vi "FGGA Serial Data Server & Recordingv4.3_10Hz.vi"(0 "VISA resource name out":refnum<visa-resource-name>, 11 "error IO":errorcluster) -> ()   [LabVIEW 2014]
uses:
  <vilib>/Instr/_visa.llb/VISA Configure Serial Port (Instr).vi
  <vilib>/Platform/TimedLoop/XDataNode/wakeup.ctl
  <vilib>/Platform/TimedLoop/XDataNode/XDNodeRunTimeDep.lvlib
  <vilib>/Platform/TimedLoop/XDataNode/nitl_modes.ctl
  <vilib>/Platform/TimedLoop/XDataNode/timing_clust.ctl
  <vilib>/platform/TimedLoop/XDataNode/XDataNode.xnode
  <vilib>/Utility/tcp.llb/UDP Multicast Write-Only Open.vi
  <vilib>/Utility/error.llb/whitespace.ctl
  C:/Program Files (x86)/National Instruments/LabVIEW 2014/examples/Data Communication/Network Streams/Simple Network Streams/support/Network Stream Command.ctl
panel:
  out "FGGA Pump":bool
  out "Flight Number":string
  out "Stop File Write":bool
  out "Default file name":string
  out "MFC":dbl[](array[numeric])
  out "FGGA restart":bool
  out "V4":bool
  out "V3":bool
  out "V2":bool
  out "V1":bool
  out "error out 2":errorcluster
  out "error out":errorcluster
  in  "MFC_1 SLPM set value":dbl
  out "Value Read":string
  out "status":bool
  in  "VISA resource name":refnum<visa-resource-name>="ASRL3::INSTR"
  in  "timeout (10sec) 2":u32=3000
  out "Labview_Viewer_UDP_Error_Out":errorcluster
  in  "Clear Display\nErrors":bool
  out "Data Processing":bool
  out "TCP Binary Packet":string
  out "UDP Time Stamp Offset":i32=1
  out "Data String":string
  out "UDP_ACSII_Out":string
  out "Serial error out":errorcluster
  out "SEPTIC TCP Error Out":errorcluster
  out "TCP packet\nSend To SEPTIC":bool
  out "FISH TCP Error Out":errorcluster
  out "TCP packet\nSend To FISH":bool
  out "UDP_Pack_num":u32
  out "UDP_Out Status":bool
  out "UDP_Out_Error Out":errorcluster
  out "Data Array":string[](array[string])
  out "RAW DATA":string
  in  "stop":bool
  out "Number of times \nRead time out":u32
  out "Loop count":i32
  # "Date"
  # "Time"
  # "CH4"
  # "CO2"
  # "H2O"
  # "Cell Pressure"
  # "Cell Temperature"
  # "Spectral Flag"
  # "Ring Down Time (Laser A)"
  # "Ring Down Time (Laser B)"
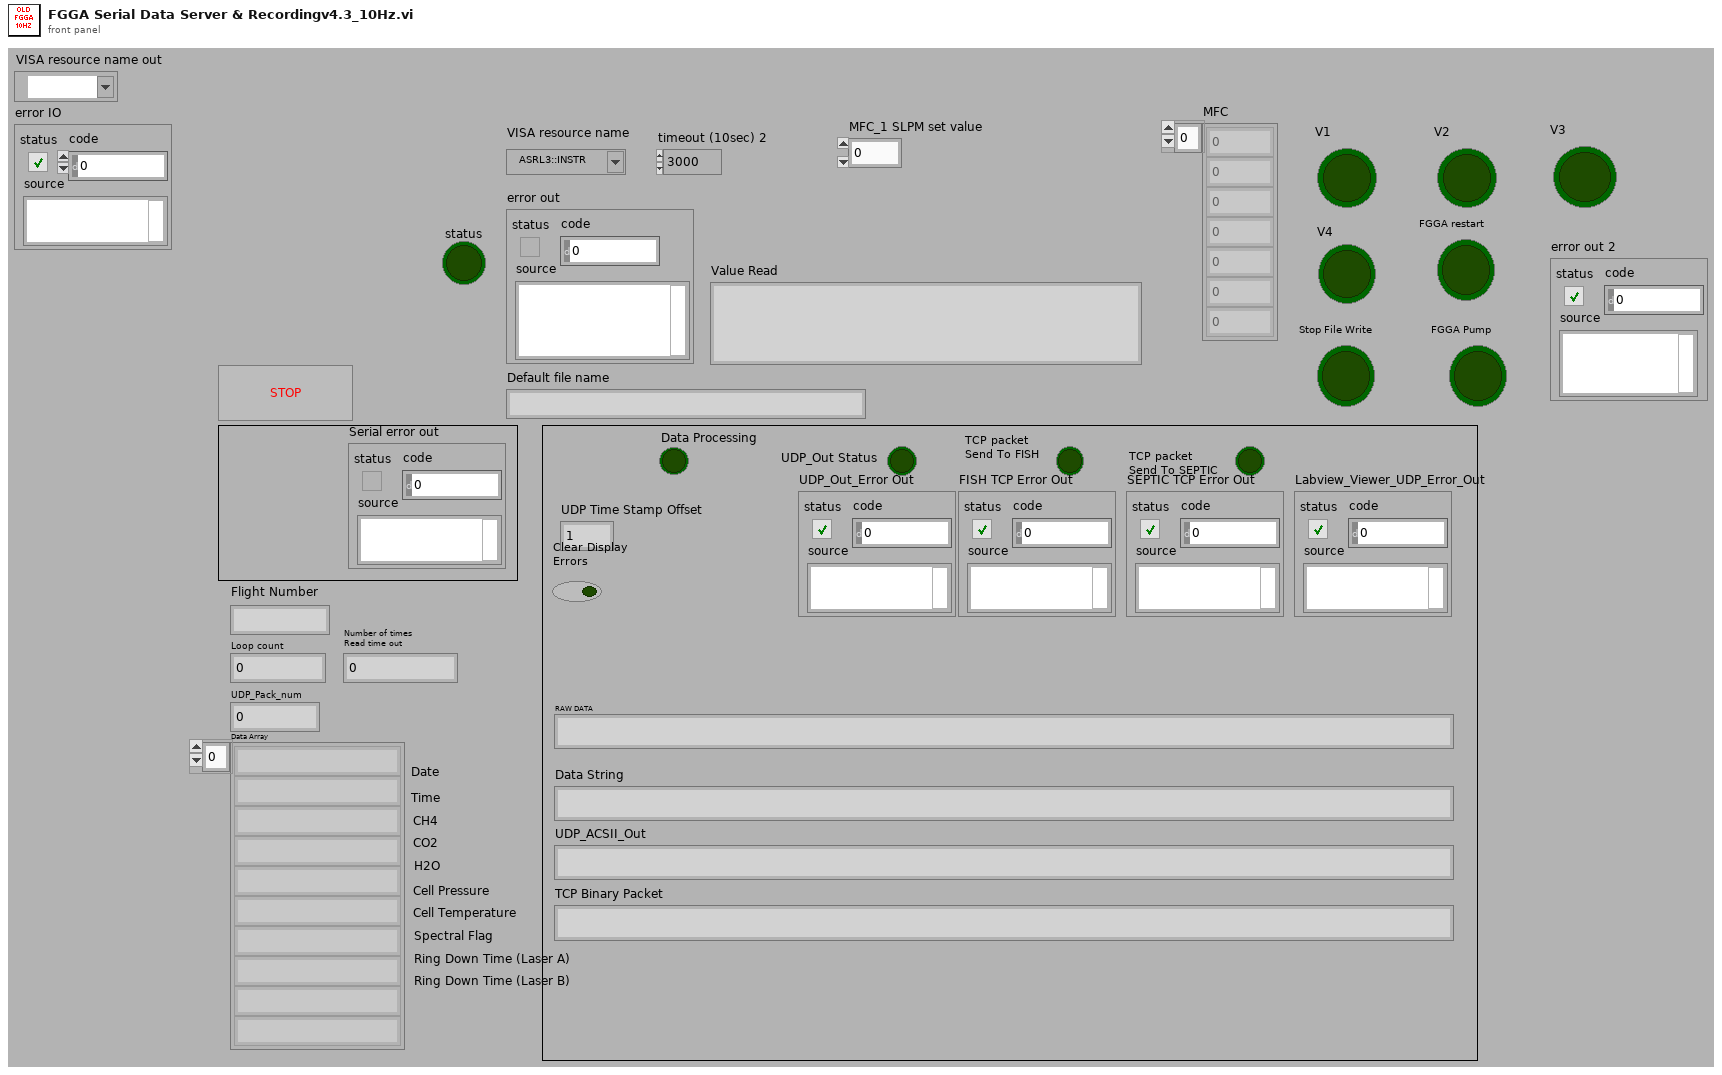
[diagram p1: front panel]
types:
  T1 = typedef "XDNodeRunTimeDep.lvlib/timing_clust.ctl" = cluster{"Expected End [f-1]":u64, "Actual End [f-1]":u64, "Finished Late? [f-1]":bool, "Expected End [i-1]":u64, "Actual End [i-1]":u64, "Finished Late? [i-1]":bool, "Expected Start [i]":u64, "Actual Start [i]":u64, "Expected Start [f]":u64, "Actual Start [f]":u64, "Source Name":string, "Structure Name":string, "Period":i64, "Deadline":i64, "Offset":i64, "Start":i64, "Priority":i32, "Timeout":i32, "Mode":T2, "Wakeup Reason":T3, "Error":errorcluster, "Source Type":string, "Secondary Source Type":string, "Global End Time":u64, "Global Start Time":u64, "Frame Duration":u64, "Iteration Duration":u64, "Assigned CPU":i32, "I/O Scan Engine Mode":u32}
  T2 = typedef "XDNodeRunTimeDep.lvlib/nitl_modes.ctl" = enum32{"No Change", "Process missed periods, maintain original phase", "Discard missed periods, maintain original phase", "Process missed periods, ignore original phase", "Discard missed periods, ignore original phase"}
  T3 = typedef "XDNodeRunTimeDep.lvlib/wakeup.ctl" = enum32{"Normal", "Aborted", "Asynchronous wakeup", "Timing source error", "Timed loop error", "Timeout"}
  T4 = typedef "Network Stream Command.ctl" = cluster{"Message":string, "Message Data":variant}
  T5 = enum16{"open", "replace", "create", "open or create", "replace or create", "replace or create with confirmation"}
  T6 = typedef "whitespace.ctl" = u16
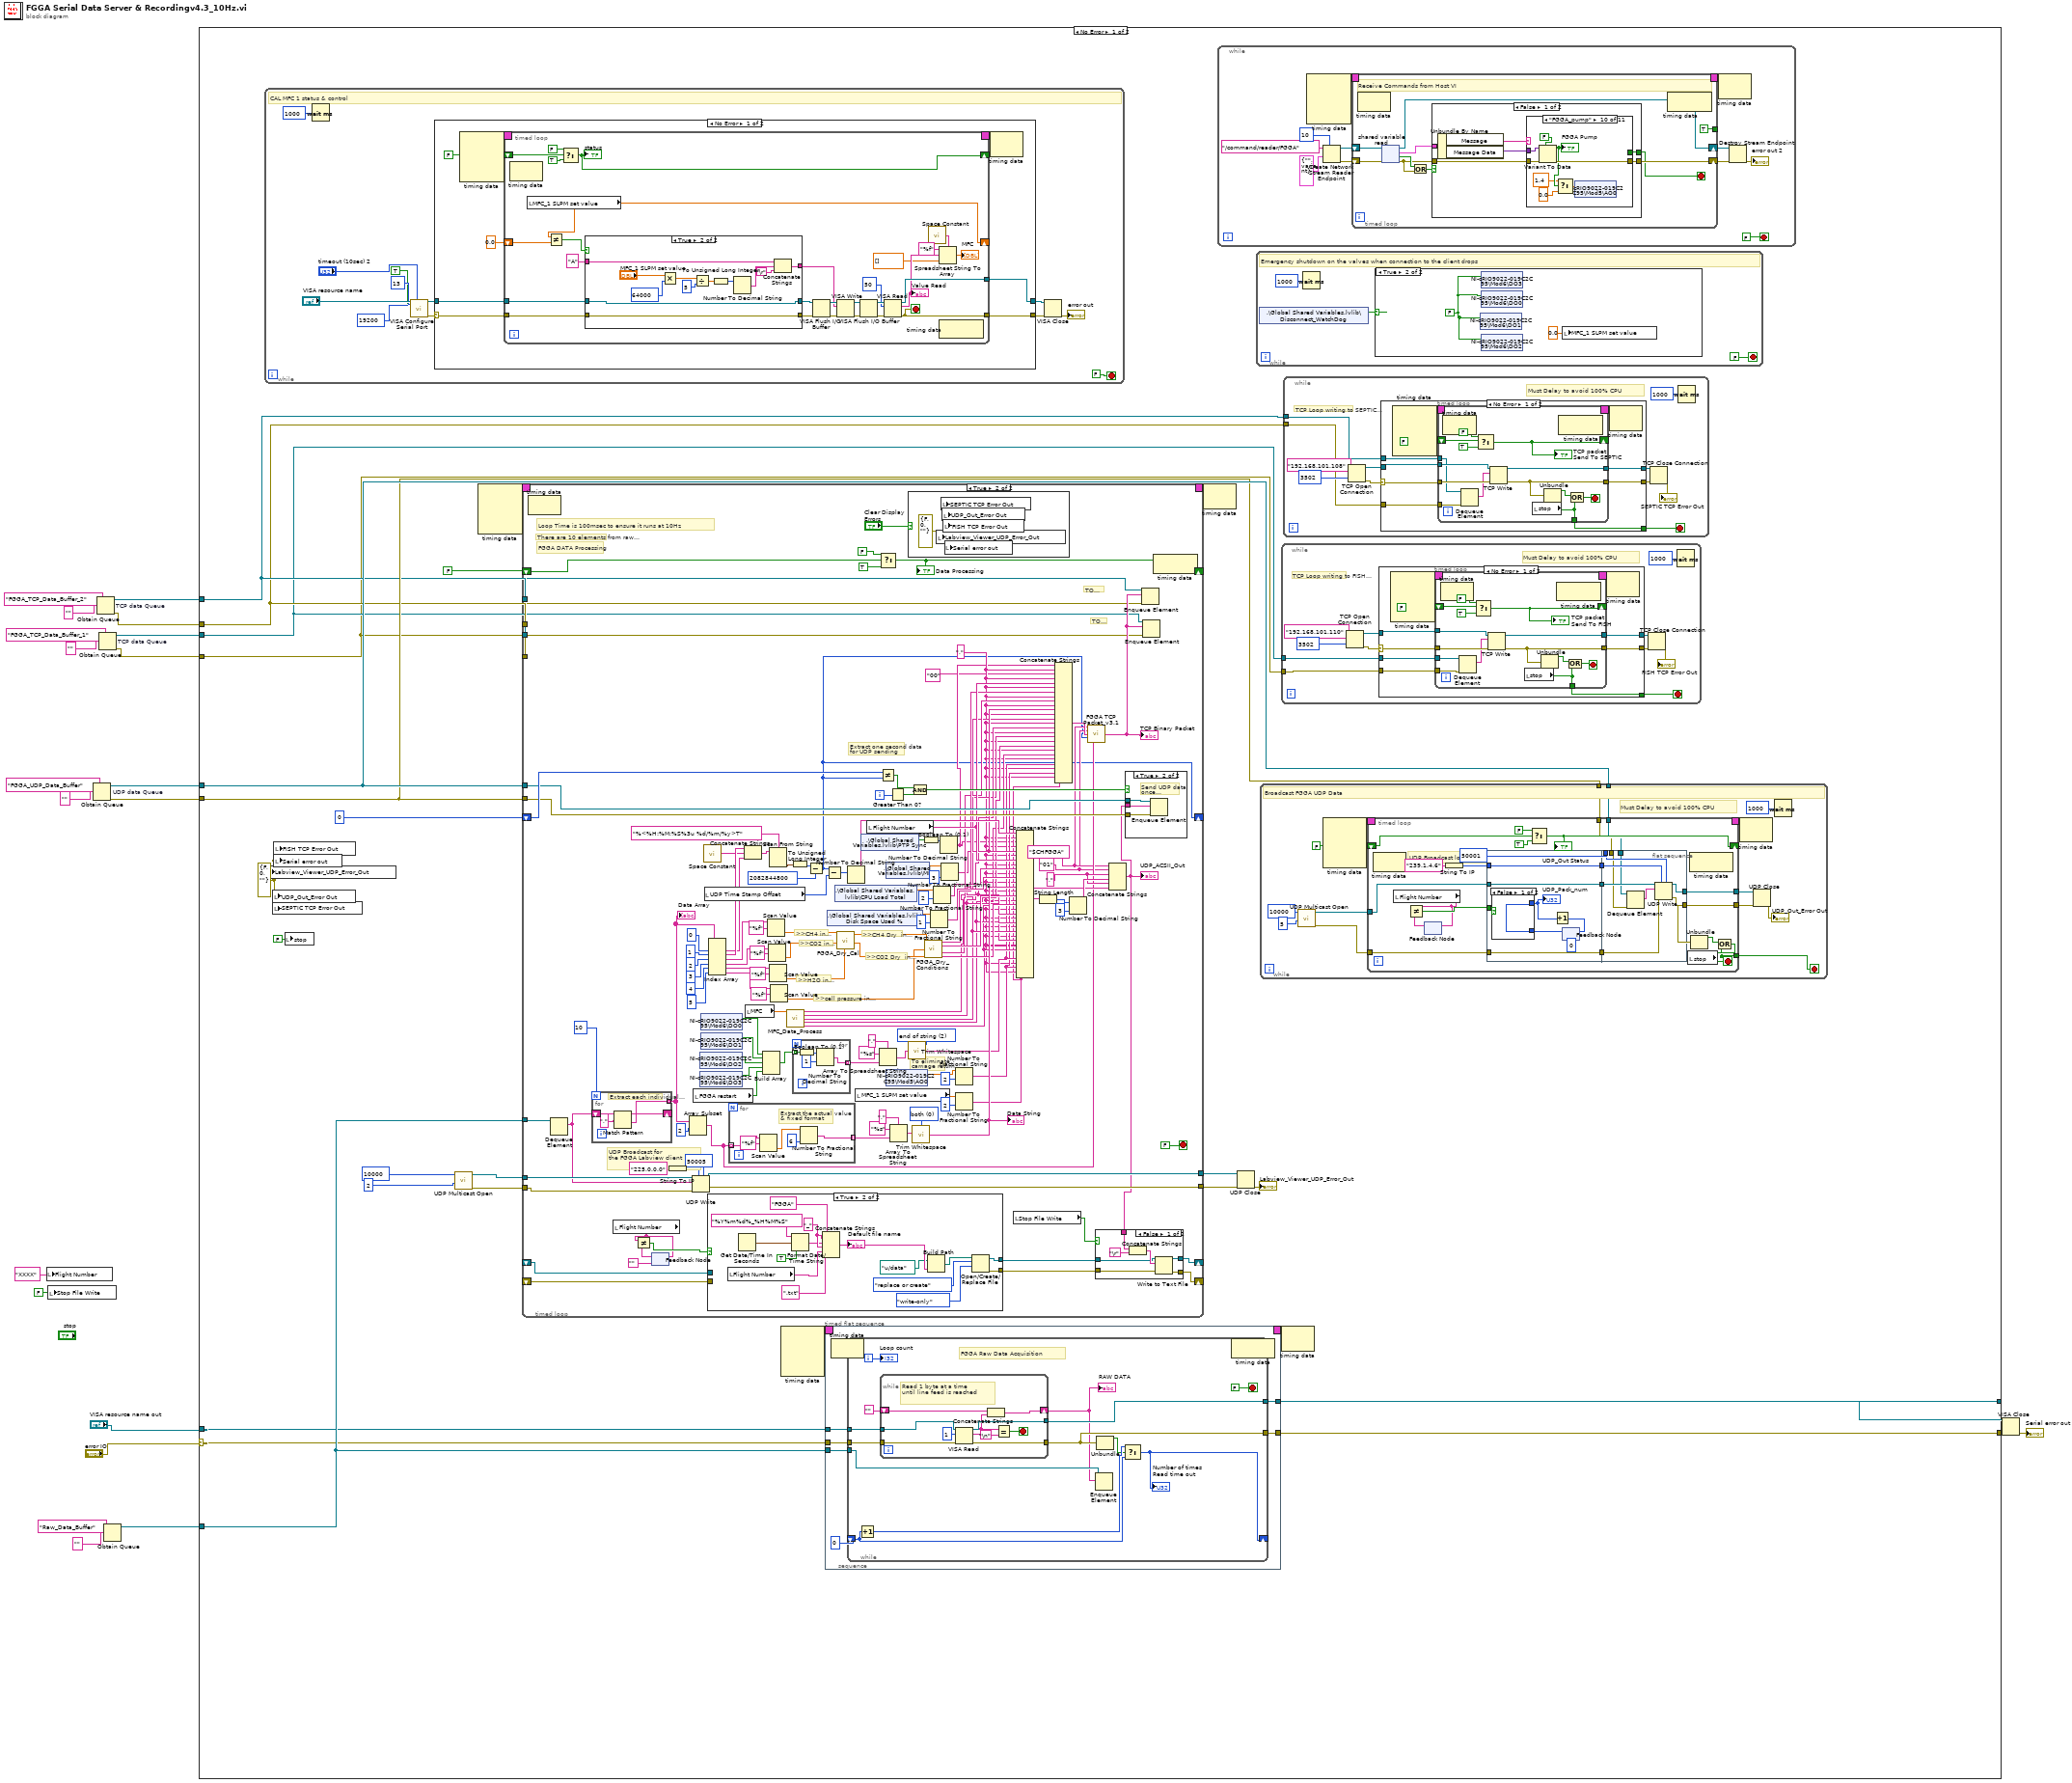
[diagram p0: block diagram]
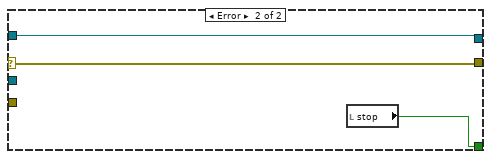
[diagram p3: hidden frame]
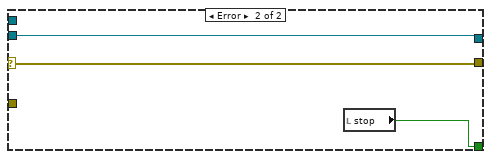
[diagram p4: hidden frame]
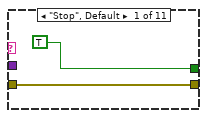
[diagram p5: hidden frame]
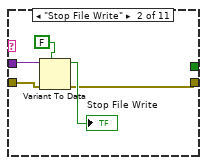
[diagram p6: hidden frame]
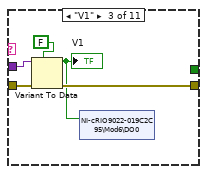
[diagram p7: hidden frame]
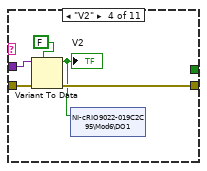
[diagram p8: hidden frame]
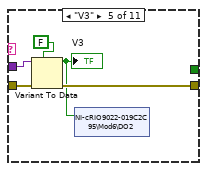
[diagram p9: hidden frame]
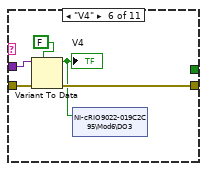
[diagram p10: hidden frame]
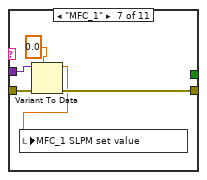
[diagram p11: hidden frame]
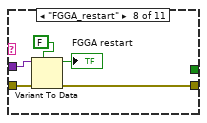
[diagram p12: hidden frame]
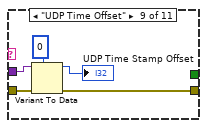
[diagram p13: hidden frame]
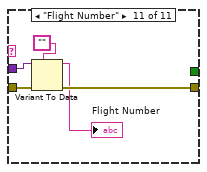
[diagram p14: hidden frame]
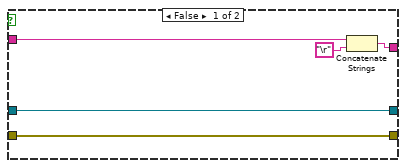
[diagram p16: hidden frame]
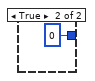
[diagram p18: hidden frame]
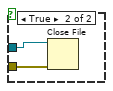
[diagram p20: hidden frame]
diagram:
  n1 = local write "Flight Number"("XXXX" ("Flight Number")) -> ()
  n2 = local write "Stop File Write"(FALSE ("Stop File Write")) -> ()
  n3 = Obtain Queue "UDP data Queue"(name (unnamed)="FGGA_UDP_Data_Buffer", element data type="") -> (queue out=w14:refnum<queue>, error out=w13:errorcluster)  [unwired: 3 in, 1 out]
  n4 = Obtain Queue "TCP data Queue"(name (unnamed)="FGGA_TCP_Data_Buffer_2", element data type="") -> (queue out=w8:refnum<queue>, error out=w7:errorcluster)  [unwired: 3 in, 1 out]
  n5 = Obtain Queue "TCP data Queue"(name (unnamed)="FGGA_TCP_Data_Buffer_1", element data type="") -> (queue out=w6:refnum<queue>, error out=w5:errorcluster)  [unwired: 3 in, 1 out]
  n6 = Obtain Queue(name (unnamed)="Raw_Data_Buffer", element data type="") -> (queue out=w20:refnum<queue>)  [unwired: 3 in, 2 out]
  n7 = case shown="No Error" "error IO" {
    selector: "error IO" -> [w25 w572]
    tunnel: "VISA resource name out" -> [w26 w573]
    tunnel: [w47 w573] -> w17
    tunnel: [w48 w572] -> w18
    tunnel: w20 -> [w44 _]
    tunnel: w14 -> [w42 _]
    tunnel: w13 -> [w41 _]
    tunnel: w8 -> [w40 _]
    tunnel: w7 -> [w39 _]
    tunnel: w6 -> [w38 _]
    tunnel: w5 -> [w37 _]
    frame No Error {
      w28 = errorcluster {"status"=FALSE, "code"=0, "source"=""} ("UDP Error Out")
      n8 = while {
        stop <- FALSE stop-if-true
        # "CAL MFC 1 status & control"
        n9 = Wait (ms)(milliseconds to wait=u32 1000) -> ()  [unwired: 1 out]
        n10 = call-poly "VISA Configure Serial Port"("VISA resource name"="VISA resource name", "timeout (10sec)"="timeout (10sec) 2", "termination char\n(0xA = '\\n' = LF)"=u8 13 ("termination char\n(0xA = '\\n' = LF)"), "Enable Termination\nChar (T)"=TRUE ("Enable Termination\nChar (T)"), "baud rate (9600)"=u32 19200) -> ("VISA resource name out"=w275:refnum<visa-resource-name>, "error out"=w271:errorcluster)  [unwired: 9 in]
        n11 = case shown="No Error" w271 {
          selector: w271 -> [w282 w332]
          tunnel: w275 -> [w283 w333]
          tunnel: [w281 w333] -> w274
          tunnel: [w280 w332] -> w273
          frame No Error {
            n12 = node-c288() -> (w278:T1)  [unwired: 4 in]
            n13 = timed-loop {
              tunnel: w283 -> [w306]
              tunnel: w282 -> [w304]
              tunnel: [w297] -> w281
              tunnel: [w292] -> w280
              shift-right: [w293] -> _
              shift-left: FALSE -> [w296]
              timing: w278 -> [_]
              timing-out: [_] -> w277
              shift-right: [w284] -> _
              shift-left: 0.0 -> [w286]
              stop <- w292 stop-if-true
              n14 = node-c288() -> ()  [unwired: 1 in, 1 out]
              n15 = local read "MFC_1 SLPM set value"() -> (w284:dbl)
              n16 = Not Equal?(x=w284, y=w286) -> (x != y?=w285:bool)
              n17 = Select(t=FALSE, s=w296, f=TRUE) -> (s? t:f=w293:bool)
              "status" <- w293
              n18 = case shown="True" w285 {
                tunnel: w306 -> [w314 w329]
                tunnel: [w314 w329] -> w305
                tunnel: w304 -> [w313 w328]
                tunnel: [w313 w328] -> w303
                tunnel: "A" -> [w317 w321]
                tunnel: [w315 w318] -> w301
                frame False {
                  n19 = Concatenate Strings(w317, "\r") -> (w315:string)
                }
                frame True {
                  n20 = Multiply(x="MFC_1 SLPM set value", y=u32 64000) -> (x*y=w325:dbl)
                  n21 = Divide(x=w325, y=u32 5) -> (x/y=w323:dbl)
                  n22 = To Unsigned Long Integer(number=w323) -> (unsigned 32bit integer=w322:u32)
                  n23 = Number To Decimal String(number=w322) -> (decimal integer string=w320:string)  [unwired: 1 in]
                  n24 = Concatenate Strings(w321, w320, "\r") -> (w318:string)
                }
              }
              n25 = VISA Flush I/O Buffer(VISA resource name=w305, error in (no error)=w303) -> (VISA resource name out=w308:refnum<visa-resource-name>, error out=w307:errorcluster)  [unwired: 1 in]
              n26 = VISA Write(VISA resource name=w308, write buffer=w301, error in (no error)=w307) -> (VISA resource name out=w300:refnum<visa-resource-name>, error out=w299:errorcluster)  [unwired: 1 out]
              n27 = VISA Flush I/O Buffer(VISA resource name=w300, error in (no error)=w299) -> (VISA resource name out=w310:refnum<visa-resource-name>, error out=w309:errorcluster)  [unwired: 1 in]
              n28 = VISA Read(VISA resource name=w310, byte count=u32 50, error in (no error)=w309) -> (VISA resource name out=w297:refnum<visa-resource-name>, read buffer=w291:string, error out=w292:errorcluster)  [unwired: 1 out]
              "Value Read" <- w291
              n29 = call <vilib>:"Space Constant.vi"() -> ("String"=w290:string)
              n30 = Spreadsheet String To Array(delimiter (Tab)=w290, format string="%f", spreadsheet string=w291, array type (2D Dbl)=dbl[] []) -> (array=→"MFC":dbl[])
              n31 = node-c288() -> ()  [unwired: 1 in, 1 out]
            }
            n32 = node-c288(w277) -> ()  [unwired: 1 out]
          }
          frame Error {
          }
        }
        n33 = VISA Close(VISA resource name=w274, error in (no error)=w273) -> (error out=→"error out":errorcluster)
      }
      n34 = local write "Labview_Viewer_UDP_Error_Out"(w28) -> ()
      n35 = local write "UDP_Out_Error Out"(w28) -> ()
      n36 = local write "SEPTIC TCP Error Out"(w28) -> ()
      n37 = local write "FISH TCP Error Out"(w28) -> ()
      n38 = local write "Serial error out"(w28) -> ()
      n39 = local write "stop"(FALSE ("stop")) -> ()
      n40 = call-poly <vilib>:"UDP Multicast Open.vi"("time-to-live (1)"=u16 2, "port"=u16 10000) -> ("error out"=w32:errorcluster, "connection ID"=w33:refnum<k16>)  [unwired: 8 in]
      n41 = node-c288() -> (w46:T1)  [unwired: 4 in]
      n42 = timed-loop {
        timing: w46 -> [_]
        timing-out: [_] -> w45
        tunnel: w44 -> [w524]
        tunnel: w42 -> [w480]
        tunnel: w41 -> [w479]
        shift-right: [w393] -> _
        shift-left: u32 0 -> [w483]
        tunnel: w40 -> [w476]
        tunnel: w39 -> [w475]
        tunnel: w38 -> [w474]
        tunnel: w37 -> [w473]
        shift-right: [w469] -> _
        shift-left: FALSE -> [w472]
        tunnel: w33 -> [w465]
        tunnel: w32 -> [w464]
        tunnel: [w463] -> w31
        tunnel: [w462] -> w30
        shift-right: [w449] -> _
        shift-left: _ -> [w441]
        shift-right: [w439] -> _
        shift-left: _ -> [w440]
        i -> [w482]
        stop <- FALSE stop-if-true
        w413 = T6 2 items=["both", "start of string", "end of string"] ("location (both)")
        w400 = ","
        w510 = T6 0 items=["both", "start of string", "end of string"] ("location (both)")
        w518 = ","
        w394 = "01"
        w395 = "$CHFGGA"
        # "To eliminate\ncarriage return"
        # ">>cell pressure in torr>>"
        # "UDP Broadcast for\nthe FGGA Labview client"
        # "There are 10 elements from raw packet"
        # "TO SEPTIC"
        # "TO FISH"
        # "Extract one second data\nfor UDP sending"
        # ">>CO2 Dry  in ppm>>"
        # ">>CH4 Dry  in ppb>>"
        # ">>H2O in ppm>>"
        # ">>CO2 in ppm>>"
        # ">>CH4 in ppm>>"
        # "Loop Time is 100msec to ensure it runs at 10Hz"
        # "FGGA DATA Processing"
        n43 = node-c288() -> ()  [unwired: 1 in, 1 out]
        n44 = Dequeue Element(queue=w524) -> (element=w461:string)  [unwired: 2 in, 3 out]
        n45 = for {
          N: 10 -> [_]
          shift-right: [w566] -> _
          shift-left: w461 -> [w564]
          tunnel: [w565] -> w515 mode=indexing
          # "Extract each individual param"
          n46 = Match Pattern(string=w564, regular expression=",") -> (before substring=w565:string, after substring=w566:string)  [unwired: 1 in, 2 out]
        }
        "Data Array" <- w515
        n47 = local read "Flight Number"() -> (w438:string)
        n48 = feedback #1("" ("Flight Number")) -> (w446:string)
        n49 = Not Equal?(x=w438, y=w446) -> (x != y?=w444:bool)
        n50 = feedback-in #1(w438) -> ()
        n51 = String To IP(1:"225.0.0.0" ("name")) -> (0:w466:u32)
        n52 = Array Subset(array=w515, index=2) -> (w478:string[])  [unwired: 1 in]
        n53 = UDP Write(address=w466, port or service name=u16 50005, connection ID=w465, data in=w461, 8:w464) -> (error out=w462:errorcluster, 3:w463:refnum<k16>)  [unwired: 1 in]
        n54 = local read "FGGA restart"() -> (w423:bool)
        n55 = shared-variable "NI-cRIO9022-019C2C95\\Mod6\\DO2"() -> (w429:bool)  [unwired: 1 in, 1 out]
        n56 = shared-variable "NI-cRIO9022-019C2C95\\Mod6\\DO3"() -> (w428:bool)  [unwired: 1 in, 1 out]
        n57 = shared-variable "NI-cRIO9022-019C2C95\\Mod6\\DO0"() -> (w431:bool)  [unwired: 1 in, 1 out]
        n58 = shared-variable "NI-cRIO9022-019C2C95\\Mod6\\DO1"() -> (w430:bool)  [unwired: 1 in, 1 out]
        n59 = call <vilib>:"Space Constant.vi"() -> ("String"=w493:string)
        n60 = local read "UDP Time Stamp Offset"() -> (w412:i32)
        n61 = case shown="True" w444 {
          tunnel: [w530 w532] -> w443
          tunnel: [w529 w531] -> w442
          tunnel: w441 -> [w530 _]
          tunnel: w440 -> [w529 _]
          frame False {
          }
          frame True {
            w538 = "_" ("string")
            n62 = local read "Flight Number"() -> (w545:string)
            n63 = Get Date/Time In Seconds() -> (seconds since 1Jan1904=w533:timestamp)
            n64 = Format Date/Time String(time format string (%c)="%Y%m%d%_%H%M%S", seconds (now)=w533, UTC format=TRUE) -> (date/time string=w535:string)
            n65 = Concatenate Strings("FGGA" ("string"), w538, w535, w538, w545, ".txt" ("string")) -> (w540:string)
            "Default file name" <- w540
            n66 = Build Path(base path=path "u:/data", name or relative path=w540) -> (appended path=w544:path)
            n67 = Open/Create/Replace File(file path (use dialog)=w544, operation (0:open)=T5."replace or create", access (0:read/write)=enum16{"read/write", "read-only", "write-only"}."write-only") -> (refnum out=w532:refnum<file>, error out=w531:errorcluster)  [unwired: 3 in, 1 out]
          }
        }
        n68 = Index Array(array=w515, index #1=0 ("index"), index #2=1 ("index"), index #3=2 ("index"), index #4=3 ("index"), index #5=4 ("index"), index #6=5 ("index")) -> (element #1=w492:string, element #2=w494:string, element #3=w498:string, element #4=w497:string, element #5=w496:string, element #6=w454:string)
        n69 = for {
          tunnel: w478 -> [w562] mode=indexing
          tunnel: [w559] -> w508 mode=indexing
          # "Extract the actual value\n& fixed format"
          n70 = Scan Value(string=w562, format string="%f") -> (value=w560:dbl)  [unwired: 1 in, 1 out]
          n71 = Number To Fractional String(number=w560, precision (6)=i16 6) -> (F-format string=w559:string)  [unwired: 2 in]
        }
        n72 = Concatenate Strings(w494, w493, w492) -> (w491:string)
        n73 = local read "MFC"() -> (w450:dbl[])
        n74 = Build Array(w431, w430, w429, w428, w423) -> (w427:bool[])
        n75 = Scan Value(string=w498, format string="%f") -> (value=w500:dbl)  [unwired: 1 in, 1 out]
        n76 = Scan Value(string=w497, format string="%f") -> (value=w499:dbl)  [unwired: 1 in, 1 out]
        n77 = Scan From String(format string="%<%H:%M:%S%3u %d/%m/%y>T", input string=w491) -> (output 1=w488:timestamp)  [unwired: 3 in, 3 out]
        n78 = Scan Value(string=w496, format string="%f") -> (value=w451:dbl)  [unwired: 1 in, 1 out]
        n79 = Scan Value(string=w454, format string="%f") -> (value=w452:dbl)  [unwired: 1 in, 1 out]
        n80 = call "MFC_Data_Process.vi"("MFC"=w450) -> ("MFC Absolute Pressure"=w407:string, "MFC Temperature"=w406:string, "MFC Volumetric Flow"=w405:string, "MFC Mass Flow"=w404:string, "MFC Set Point"=w403:string)  [unwired: 10 in]
        n81 = To Unsigned Long Integer(number=w488) -> (unsigned 32bit integer=w489:u32)
        n82 = for {
          tunnel: w427 -> [w527] mode=indexing
          tunnel: [w526] -> w424 mode=indexing
          n83 = Boolean To (0,1)(Boolean=w527) -> (0, 1=w528:i16)
          n84 = Number To Decimal String(number=w528, width (-)=i16 1) -> (decimal integer string=w526:string)
        }
        n85 = Subtract(x=w489, y=u32 2082844800) -> (x-y=w393:u32)
        n86 = Subtract(x=w393, y=w412) -> (x-y=w486:u32)
        n87 = shared-variable ".\\Global Shared Variables.lvlib\\Disk Space Used %"() -> (w416:dbl)  [unwired: 1 in, 1 out]
        n88 = shared-variable ".\\Global Shared Variables.lvlib\\CPU Load Total"() -> (w437:dbl)  [unwired: 1 in, 1 out]
        n89 = call "FGGA_Dry_Cal.vi"("H2O"=w451, "CO2_Wet"=w499, "CH4_Wet"=w500) -> ("CO2_Dry"=w456:dbl, "CH4_Dry"=w458:dbl)  [unwired: 7 in]
        n90 = Number To Decimal String(number=w486) -> (decimal integer string=w487:string)  [unwired: 1 in]
        n91 = local read "MFC_1 SLPM set value"() -> (w419:dbl)
        n92 = shared-variable ".\\Global Shared Variables.lvlib\\PTP Sync"() -> (w432:bool)  [unwired: 1 in, 1 out]
        n93 = local read "Flight Number"() -> (w411:string)
        n94 = Array To Spreadsheet String(delimiter (Tab)=",", array=w424, 3:"%s" ("format string")) -> (spreadsheet string=w414:string)
        n95 = Select(t=FALSE, s=w472, f=TRUE) -> (s? t:f=w469:bool)
        "Data Processing" <- w469
        n96 = Not Equal?(x=w483, y=w393) -> (x != y?=w484:bool)
        n97 = shared-variable ".\\Global Shared Variables.lvlib\\MFM"() -> (w435:dbl)  [unwired: 1 in, 1 out]
        n98 = shared-variable "NI-cRIO9022-019C2C95\\Mod5\\AO0"() -> (w421:dbl)  [unwired: 1 in, 1 out]
        n99 = Greater Than 0?(x=w482) -> (x > 0?=w485:bool)
        n100 = Array To Spreadsheet String(delimiter (Tab)=",", array=w508, 3:"%s" ("format string")) -> (spreadsheet string=w509:string)
        n101 = case shown="True" "Clear Display\nErrors" {
          frame False {
          }
          frame True {
            w555 = errorcluster {"status"=FALSE, "code"=0, "source"=""} ("UDP Error Out")
            n102 = local write "Labview_Viewer_UDP_Error_Out"(w555) -> ()
            n103 = local write "SEPTIC TCP Error Out"(w555) -> ()
            n104 = local write "UDP_Out_Error Out"(w555) -> ()
            n105 = local write "FISH TCP Error Out"(w555) -> ()
            n106 = local write "Serial error out"(w555) -> ()
          }
        }
        n107 = call <vilib>:"Trim Whitespace.vi"("string"=w414, "location (both)"=w413) -> ("trimmed string"=w402:string)
        n108 = call <vilib>:"Trim Whitespace.vi"("string"=w509, "location (both)"=w510) -> ("trimmed string"=w507:string)
        "Data String" <- w507
        n109 = Compound Arithmetic op=AND(w484, w485) -> (w481:bool)
        n110 = Boolean To (0,1)(Boolean=w432) -> (0, 1=w433:i16)
        n111 = call "FGGA_Dry_Conditions.vi"("CH4_Dry"=w458, "Pressure"=w452, "CO2_Dry"=w456) -> ("CH4_Dry_TCP"=w410:string, "CH4_Dry_UDP"=w460:string, "CO2_Dry_TCP"=w409:string, "CO2_Dry_UDP"=w459:string)  [unwired: 9 in]
        n112 = Number To Fractional String(number=w416, precision (6)=i16 1) -> (F-format string=w415:string)  [unwired: 2 in]
        n113 = Number To Fractional String(number=w437, precision (6)=i16 2) -> (F-format string=w418:string)  [unwired: 2 in]
        n114 = Number To Decimal String(number=w433) -> (decimal integer string=w397:string)  [unwired: 1 in]
        n115 = Number To Fractional String(number=w435, precision (6)=i16 3) -> (F-format string=w408:string)  [unwired: 2 in]
        n116 = Number To Fractional String(number=w421, precision (6)=i16 2) -> (F-format string=w401:string)  [unwired: 2 in]
        n117 = Number To Fractional String(number=w419, precision (6)=i16 2) -> (F-format string=w399:string)  [unwired: 2 in]
        n118 = local read "Stop File Write"() -> (w447:bool)
        n119 = Concatenate Strings(w487, w400, w397, w400, w408, w400, w411, w400, w418, w400, w415, w400, w507, w400, w460, w400, w459, w400, w407, w400, w406, w400, w405, w400, w404, w400, w403, w400, w402, w400, w401, w400, w399) -> (w517:string)
        n120 = String Length(string=w517) -> (length=w521:i32)
        n121 = Concatenate Strings(w397, w400, "00", w400, w411, w400, w410, w400, w409, w400, w408, w400, w407, w400, w406, w400, w405, w400, w404, w400, w403, w400, w402, w400, w401, w400, w399) -> (w398:string)
        n122 = Number To Decimal String(number=w521, width (-)=i16 3) -> (decimal integer string=w519:string)
        n123 = call "FGGA TCP Packet_v3.1.vi"("ID"=w395, "Version"=w394, "TCP Packet In"=w398, "utc_time"=w393, "Data Array"=w478) -> ("TCP Binary Packet"=w477:string)  [unwired: 10 in]
        "TCP Binary Packet" <- w477
        n124 = Concatenate Strings(w395, w394, w518, w519, w518, w517) -> (w448:string)
        "UDP_ACSII_Out" <- w448
        n125 = case shown="False" w447 {
          tunnel: w448 -> [w552 _]
          tunnel: [w549 _] -> w449
          tunnel: w443 -> [w548 w554]
          tunnel: w442 -> [w547 w553]
          tunnel: [w546 _] -> w439
          frame False {
            n126 = Concatenate Strings(w552, "\r") -> (w550:string)
            n127 = Write to Text File(file (use dialog)=w548, text=w550, error in=w547) -> (refnum out=w549:refnum<file>, error out=w546:errorcluster)  [unwired: 2 out]
          }
          frame True {
            n128 = Close File(refnum=w554, error in=w553) -> ()  [unwired: 2 out]
          }
        }
        n129 = case shown="True" w481 {
          tunnel: w448 -> [_ w558]
          tunnel: w480 -> [_ w557]
          tunnel: w479 -> [_ w556]
          frame False {
          }
          frame True {
            # "Send UDP data once\na second"
            n130 = Enqueue Element(queue=w557, element=w558, error in (no error)=w556) -> ()  [unwired: 1 in, 3 out]
          }
        }
        n131 = Enqueue Element(queue=w476, element=w477, error in (no error)=w475) -> ()  [unwired: 1 in, 3 out]
        n132 = Enqueue Element(queue=w474, element=w477, error in (no error)=w473) -> ()  [unwired: 1 in, 3 out]
        n133 = node-c288() -> ()  [unwired: 1 in, 1 out]
      }
      n134 = node-c288() -> (w24:T1)  [unwired: 4 in]
      n135 = timed-sequence {
        timing: w24 -> [_]
        timing-out: [_] -> w23
        tunnel: [w142] -> w48
        tunnel: [w141] -> w47
        tunnel: w44 -> [w140]
        tunnel: w26 -> [w139]
        tunnel: w25 -> [w138]
        n136 = timed-flat-sequence {
          tunnel: [w148] -> w142
          tunnel: [w147] -> w141
          tunnel: w140 -> [w145]
          tunnel: w139 -> [w144]
          tunnel: w138 -> [w143]
          n137 = node-c288() -> ()  [unwired: 1 in, 1 out]
          n138 = while {
            tunnel: w144 -> [w161]
            tunnel: w143 -> [w160]
            tunnel: [w159] -> w148
            shift-right: [w155] -> _
            shift-left: u32 0 -> [w156]
            tunnel: [w158] -> w147
            tunnel: w145 -> [w152]
            i -> [w157]
            stop <- FALSE stop-if-true
            # "FGGA Raw Data Acquisition"
            n139 = Increment(x=w156) -> (x+1=w154:u32)
            n140 = while {
              tunnel: [w171] -> w158
              tunnel: [w170] -> w159
              tunnel: w161 -> [w169]
              tunnel: w160 -> [w168]
              shift-right: [w166] -> w151
              shift-left: "" -> [w167]
              stop <- w163 stop-if-true
              # "Read 1 byte at a time \nuntil line feed is reached"
              n141 = VISA Read(VISA resource name=w169, byte count=u32 1, error in (no error)=w168) -> (VISA resource name out=w171:refnum<visa-resource-name>, read buffer=w165:string, error out=w170:errorcluster)  [unwired: 1 out]
              n142 = Concatenate Strings(w167, w165) -> (w166:string)
              n143 = Equal?(x=w165, y="\n") -> (x = y?=w163:bool)
            }
            "RAW DATA" <- w151
            n144 = Enqueue Element(queue=w152, element=w151) -> ()  [unwired: 2 in, 3 out]
            n145 = Unbundle(w159) -> ("status"=w150:bool)  [unwired: 2 out]
            n146 = Select(t=w154, s=w150, f=w156) -> (s? t:f=w155:u32)
            "Number of times \nRead time out" <- w155
            "Loop count" <- w157
          }
          n147 = node-c288() -> ()  [unwired: 1 in, 1 out]
        }
      }
      n148 = node-c288(w45) -> ()  [unwired: 1 out]
      n149 = while {
        stop <- FALSE stop-if-true
        n150 = node-c288() -> (w177:T1)  [unwired: 4 in]
        n151 = Create Network Stream Reader Endpoint(7:10 ("reader buffer size"), 9:T4 {"Message"="", "Message Data"=variant} ("Message Cluster"), 11:"/command/reader/FGGA" ("reader url")) -> (0:w182:errorcluster, 3:w183:refnum<k21>)  [unwired: 4 in]
        n152 = timed-loop "Host->Target Command Reader" {
          shift-right: [w193] -> w180
          shift-left: w182 -> [w196]
          shift-right: [w194] -> w179
          shift-left: w183 -> [w195]
          tunnel: [TRUE] -> _
          timing: w177 -> [_]
          timing-out: [_] -> w176
          stop <- w187 stop-if-true
          # "Receive Commands from Host VI"
          n153 = node-c288() -> ()  [unwired: 1 in, 1 out]
          n154 = shared-variable-read(w195, w196) -> (w194:refnum<k21>, w189:errorcluster, w191:bool, w192:T4)  [unwired: 1 in]
          n155 = Or(x=w191, y=w189) -> (x .or. y?=w190:bool)
          n156 = case shown="False" w190 {
            selector: w190 -> [_ w260]
            tunnel: w189 -> [w204 w261]
            tunnel: [w203 w261] -> w193
            tunnel: w192 -> [w201 _]
            tunnel: [w202 w260] -> w187
            frame False {
              n157 = Unbundle By Name(w201) -> ("Message"=w200:string, "Message Data"=w199:variant)
              n158 = case shown="\"FGGA_pump\"" w200 {
                tunnel: w204 -> [w206 w211 w216 w221 w226 w231 w236 w241 w246 w254 w259]
                tunnel: [w206 w207 w215 w220 w225 w230 w235 w240 w245 w253 w258] -> w203
                tunnel: w199 -> [_ w210 w214 w219 w224 w229 w234 w239 w244 w252 w257]
                tunnel: [TRUE _ _ _ _ _ _ _ _ _ _] -> w202
                frame "Stop", Default {
                }
                frame "Stop File Write" {
                  n159 = Variant To Data(error in=w211, type=FALSE, Variant=w210) -> (data=→"Stop File Write":bool, error out=w207:errorcluster)
                }
                frame "V1" {
                  n160 = Variant To Data(error in=w216, type=FALSE, Variant=w214) -> (data=w212:bool, error out=w215:errorcluster)
                  "V1" <- w212
                  n161 = shared-variable "NI-cRIO9022-019C2C95\\Mod6\\DO0"(w212) -> ()  [unwired: 1 in, 1 out]
                }
                frame "V2" {
                  n162 = Variant To Data(error in=w221, type=FALSE, Variant=w219) -> (data=w217:bool, error out=w220:errorcluster)
                  "V2" <- w217
                  n163 = shared-variable "NI-cRIO9022-019C2C95\\Mod6\\DO1"(w217) -> ()  [unwired: 1 in, 1 out]
                }
                frame "V3" {
                  n164 = Variant To Data(error in=w226, type=FALSE, Variant=w224) -> (data=w222:bool, error out=w225:errorcluster)
                  "V3" <- w222
                  n165 = shared-variable "NI-cRIO9022-019C2C95\\Mod6\\DO2"(w222) -> ()  [unwired: 1 in, 1 out]
                }
                frame "V4" {
                  n166 = Variant To Data(error in=w231, type=FALSE, Variant=w229) -> (data=w227:bool, error out=w230:errorcluster)
                  "V4" <- w227
                  n167 = shared-variable "NI-cRIO9022-019C2C95\\Mod6\\DO3"(w227) -> ()  [unwired: 1 in, 1 out]
                }
                frame "MFC_1" {
                  n168 = Variant To Data(error in=w236, type=0.0, Variant=w234) -> (data=w232:dbl, error out=w235:errorcluster)
                  n169 = local write "MFC_1 SLPM set value"(w232) -> ()
                }
                frame "FGGA_restart" {
                  n170 = Variant To Data(error in=w241, type=FALSE, Variant=w239) -> (data=→"FGGA restart":bool, error out=w240:errorcluster)
                }
                frame "UDP Time Offset" {
                  n171 = Variant To Data(error in=w246, type=0, Variant=w244) -> (data=→"UDP Time Stamp Offset":i32, error out=w245:errorcluster)
                }
                frame "FGGA_pump" {
                  n172 = Variant To Data(error in=w254, type=FALSE, Variant=w252) -> (data=w249:bool, error out=w253:errorcluster)
                  "FGGA Pump" <- w249
                  n173 = Select(t=1.4 ("f"), s=w249, f=0.0 ("t")) -> (s? t:f=w250:dbl)
                  n174 = shared-variable "NI-cRIO9022-019C2C95\\Mod5\\AO0"(w250) -> ()  [unwired: 1 in, 1 out]
                }
                frame "Flight Number" {
                  n175 = Variant To Data(error in=w259, type="", Variant=w257) -> (data=→"Flight Number":string, error out=w258:errorcluster)
                }
              }
            }
            frame True {
            }
          }
          n176 = node-c288() -> ()  [unwired: 1 in, 1 out]
        }
        n177 = node-c288(w176) -> ()  [unwired: 1 out]
        n178 = Destroy Stream Endpoint(8:w180, 11:w179) -> (0:→"error out 2":errorcluster)
      }
      n179 = UDP Close(connection ID=w31, 8:w30) -> (error out=→"Labview_Viewer_UDP_Error_Out":errorcluster)  [unwired: 1 out]
      n180 = while {
        stop <- FALSE stop-if-true
        # "Emergency shutdown on the valves when connection to the client drops"
        n181 = shared-variable ".\\Global Shared Variables.lvlib\\Disconnect_WatchDog"() -> (w49:bool)  [unwired: 1 in, 1 out]
        n182 = Wait (ms)(milliseconds to wait=u32 1000) -> ()  [unwired: 1 out]
        n183 = case shown="True" w49 {
          frame False {
          }
          frame True {
            w53 = FALSE
            n184 = shared-variable "NI-cRIO9022-019C2C95\\Mod6\\DO1"(w53) -> ()  [unwired: 1 in, 1 out]
            n185 = shared-variable "NI-cRIO9022-019C2C95\\Mod6\\DO3"(w53) -> ()  [unwired: 1 in, 1 out]
            n186 = shared-variable "NI-cRIO9022-019C2C95\\Mod6\\DO0"(w53) -> ()  [unwired: 1 in, 1 out]
            n187 = shared-variable "NI-cRIO9022-019C2C95\\Mod6\\DO2"(w53) -> ()  [unwired: 1 in, 1 out]
            n188 = local write "MFC_1 SLPM set value"(0.0 ("MFC_1 SLPM set value")) -> ()
          }
        }
      }
      n189 = while {
        tunnel: w42 -> [w336]
        tunnel: w41 -> [w335]
        stop <- w337 stop-if-true
        # "Must Delay to avoid 100% CPU"
        # "Broadcast FGGA UDP Data"
        n190 = call-poly <vilib>:"UDP Multicast Open.vi"("time-to-live (1)"=u16 5, "port"=u16 10000) -> ("error out"=w344:errorcluster, "connection ID"=w345:refnum<k16>)  [unwired: 8 in]
        n191 = node-c288() -> (w347:T1)  [unwired: 4 in]
        n192 = timed-loop {
          tunnel: w345 -> [w368]
          tunnel: w344 -> [w367]
          timing: w347 -> [_]
          timing-out: [_] -> w346
          shift-right: [w356] -> _
          shift-left: FALSE -> [w359]
          tunnel: [w355] -> w339
          tunnel: [w353] -> w338
          tunnel: [w351] -> w337
          tunnel: w336 -> [w349]
          tunnel: w335 -> [w348]
          stop <- w352 stop-if-true
          # "UDP Broadcast loop"
          n193 = node-c288() -> ()  [unwired: 1 in, 1 out]
          n194 = local read "Flight Number"() -> (w350:string)
          n195 = feedback-in #2(w350) -> ()
          n196 = feedback #2() -> (w361:string)  [unwired: 1 in]
          n197 = Not Equal?(x=w350, y=w361) -> (x != y?=w360:bool)
          n198 = String To IP(1:"239.1.4.6" ("name")) -> (0:w365:u32)
          n199 = flat-sequence {
            tunnel: w365 -> [w375]
            tunnel: w367 -> [w376]
            tunnel: w368 -> [w377]
            tunnel: [w377] -> w364
            tunnel: [w376] -> w363
            tunnel: [w375] -> w362
            tunnel: w360 -> [w374]
            tunnel: u16 50001 ("port or service name") -> [w388]
            tunnel: w364 -> [w387]
            tunnel: w363 -> [w386]
            tunnel: w362 -> [w385]
            tunnel: [w384] -> w355
            tunnel: [w383] -> w353
            tunnel: w349 -> [w381]
            tunnel: w348 -> [w380]
            frame #0 {
              n200 = feedback #3(u32 0) -> (w371:u32)
              n201 = case shown="False" w374 {
                tunnel: w371 -> [w378 _]
                tunnel: [w378 u32 0] -> w370
                frame False {
                }
                frame True {
                }
              }
              "UDP_Pack_num" <- w370
              n202 = Increment(x=w370) -> (x+1=w372:u32)
              n203 = feedback-in #3(w372) -> ()
            }
            frame #1 {
              n204 = Dequeue Element(queue=w381, error in (no error)=w380) -> (element=w382:string)  [unwired: 1 in, 3 out]
              n205 = UDP Write(address=w385, port or service name=w388, connection ID=w387, data in=w382, 8:w386) -> (error out=w383:errorcluster, 3:w384:refnum<k16>)  [unwired: 1 in]
            }
          }
          n206 = Select(t=FALSE, s=w359, f=TRUE) -> (s? t:f=w356:bool)
          "UDP_Out Status" <- w356
          n207 = local read "stop"() -> (w351:bool)
          n208 = node-c288() -> ()  [unwired: 1 in, 1 out]
          n209 = Unbundle(w353) -> ("status"=w354:bool)  [unwired: 2 out]
          n210 = Compound Arithmetic op=OR(w354, w351) -> (w352:bool)
        }
        n211 = node-c288(w346) -> ()  [unwired: 1 out]
        n212 = UDP Close(connection ID=w339, 8:w338) -> (error out=→"UDP_Out_Error Out":errorcluster)  [unwired: 1 out]
        n213 = Wait (ms)(milliseconds to wait=u32 1000) -> ()  [unwired: 1 out]
      }
      n214 = while {
        tunnel: w38 -> [w56]
        tunnel: w37 -> [w55]
        stop <- w59 stop-if-true
        # "Must Delay to avoid 100% CPU"
        # "TCP Loop writing to FISH Tank"
        n215 = TCP Open Connection(address="192.168.101.110", remote port or service name=u16 3502) -> (connection ID=w62:refnum<k5>, error out=w57:errorcluster)  [unwired: 3 in]
        n216 = case shown="No Error" w57 {
          selector: w57 -> [w67 w94]
          tunnel: w62 -> [w72 w95]
          tunnel: [w71 w95] -> w61
          tunnel: [w70 w94] -> w60
          tunnel: [w69 w93] -> w59
          tunnel: w56 -> [w66 _]
          tunnel: w55 -> [w65 _]
          frame No Error {
            n217 = node-c288() -> (w74:T1)  [unwired: 4 in]
            n218 = timed-loop {
              tunnel: w72 -> [w88]
              tunnel: w67 -> [w87]
              tunnel: [w86] -> w71
              tunnel: [w85] -> w70
              tunnel: [w77] -> w69
              shift-right: [w79] -> _
              shift-left: FALSE -> [w82]
              timing: w74 -> [_]
              timing-out: [_] -> w73
              tunnel: w66 -> [w76]
              tunnel: w65 -> [w75]
              stop <- w83 stop-if-true
              n219 = node-c288() -> ()  [unwired: 1 in, 1 out]
              n220 = Dequeue Element(queue=w76, error in (no error)=w75) -> (element=w78:string)  [unwired: 1 in, 3 out]
              n221 = Select(t=FALSE, s=w82, f=TRUE) -> (s? t:f=w79:bool)
              "TCP packet\nSend To FISH" <- w79
              n222 = TCP Write(connection ID=w88, data in=w78, error in (no error)=w87) -> (connection ID out=w86:refnum<k5>, error out=w85:errorcluster)  [unwired: 1 in, 1 out]
              n223 = local read "stop"() -> (w77:bool)
              n224 = Unbundle(w85) -> ("status"=w84:bool)  [unwired: 2 out]
              n225 = node-c288() -> ()  [unwired: 1 in, 1 out]
              n226 = Compound Arithmetic op=OR(w84, w77) -> (w83:bool)
            }
            n227 = node-c288(w73) -> ()  [unwired: 1 out]
          }
          frame Error {
            n228 = local read "stop"() -> (w93:bool)
          }
        }
        n229 = TCP Close Connection(connection ID=w61, error in (no error)=w60) -> (error out=→"FISH TCP Error Out":errorcluster)  [unwired: 1 in, 1 out]
        n230 = Wait (ms)(milliseconds to wait=u32 1000) -> ()  [unwired: 1 out]
      }
      n231 = node-c288(w23) -> ()  [unwired: 1 out]
      n232 = while {
        tunnel: w40 -> [w98]
        tunnel: w39 -> [w97]
        stop <- w101 stop-if-true
        # "Must Delay to avoid 100% CPU"
        # "TCP Loop writing to SEPTIC Tank"
        n233 = TCP Open Connection(address="192.168.101.108", remote port or service name=u16 3502) -> (connection ID=w104:refnum<k5>, error out=w99:errorcluster)  [unwired: 3 in]
        n234 = case shown="No Error" w99 {
          selector: w99 -> [w109 w136]
          tunnel: w104 -> [w114 w137]
          tunnel: [w113 w137] -> w103
          tunnel: [w112 w136] -> w102
          tunnel: [w111 w135] -> w101
          tunnel: w98 -> [w108 _]
          tunnel: w97 -> [w107 _]
          frame No Error {
            n235 = node-c288() -> (w116:T1)  [unwired: 4 in]
            n236 = timed-loop {
              tunnel: w114 -> [w130]
              tunnel: w109 -> [w129]
              tunnel: [w128] -> w113
              tunnel: [w127] -> w112
              tunnel: [w119] -> w111
              shift-right: [w121] -> _
              shift-left: FALSE -> [w124]
              timing: w116 -> [_]
              timing-out: [_] -> w115
              tunnel: w108 -> [w118]
              tunnel: w107 -> [w117]
              stop <- w125 stop-if-true
              n237 = node-c288() -> ()  [unwired: 1 in, 1 out]
              n238 = Dequeue Element(queue=w118, error in (no error)=w117) -> (element=w120:string)  [unwired: 1 in, 3 out]
              n239 = Select(t=FALSE, s=w124, f=TRUE) -> (s? t:f=w121:bool)
              "TCP packet\nSend To SEPTIC" <- w121
              n240 = TCP Write(connection ID=w130, data in=w120, error in (no error)=w129) -> (connection ID out=w128:refnum<k5>, error out=w127:errorcluster)  [unwired: 1 in, 1 out]
              n241 = local read "stop"() -> (w119:bool)
              n242 = Unbundle(w127) -> ("status"=w126:bool)  [unwired: 2 out]
              n243 = node-c288() -> ()  [unwired: 1 in, 1 out]
              n244 = Compound Arithmetic op=OR(w126, w119) -> (w125:bool)
            }
            n245 = node-c288(w115) -> ()  [unwired: 1 out]
          }
          frame Error {
            n246 = local read "stop"() -> (w135:bool)
          }
        }
        n247 = TCP Close Connection(connection ID=w103, error in (no error)=w102) -> (error out=→"SEPTIC TCP Error Out":errorcluster)  [unwired: 1 in, 1 out]
        n248 = Wait (ms)(milliseconds to wait=u32 1000) -> ()  [unwired: 1 out]
      }
    }
    frame Error {
    }
  }
  n249 = VISA Close(VISA resource name=w17, error in (no error)=w18) -> (error out=→"Serial error out":errorcluster)
